vi "ParseServerMessage.vi"(8 "error in (no error)":errorcluster, 10 "msg":string) -> (0 "error out":errorcluster, 2 "ServerFrame":T1)   [LabVIEW 2017, in "LabVIEW STOMP.lvlib" / "STOMP.lvclass"]
uses:
  STOMP.lvclass
  Typedefs/Type_ServerFrame.ctl
  Typedefs/Type_ServerFrameType.ctl
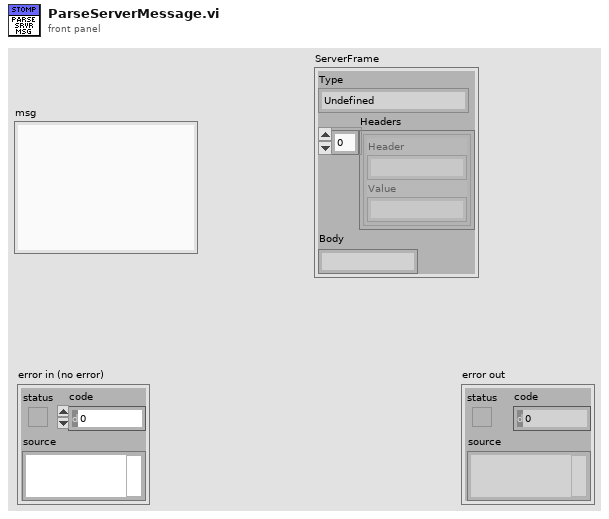
[diagram p1: front panel]
types:
  T1 = typedef "LabVIEW STOMP.lvlib/STOMP.lvclass/Type_ServerFrame.ctl" = cluster{"Type":T2, "Headers":cluster{"Header":string, "Value":string}[], "Body":string}
  T2 = typedef "LabVIEW STOMP.lvlib/STOMP.lvclass/Type_ServerFrameType.ctl" = enum16{"Undefined", "MESSAGE", "CONNECTED", "RECEIPT", "ERROR"}
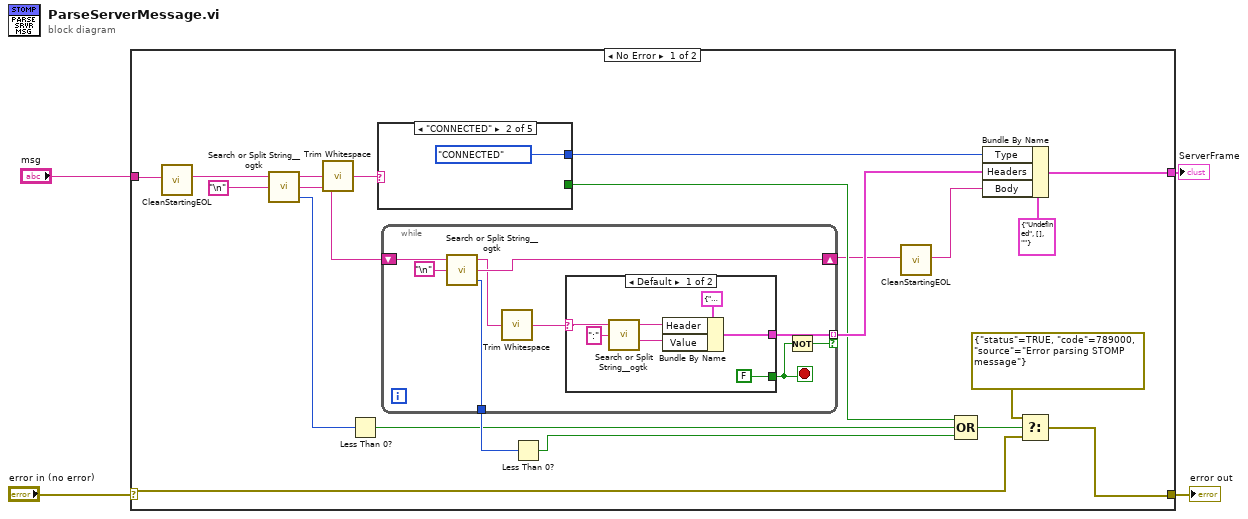
[diagram p0: block diagram]
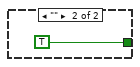
[diagram p2: hidden frame]
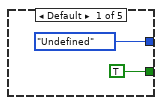
[diagram p3: hidden frame]
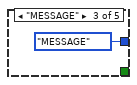
[diagram p4: hidden frame]
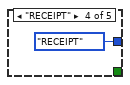
[diagram p5: hidden frame]
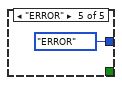
[diagram p6: hidden frame]
diagram:
  n1 = case shown="No Error" "error in (no error)" {
    selector: "error in (no error)" -> [w11 w49]
    tunnel: [w10 w49] -> w3
    tunnel: "msg" -> [w8 _]
    tunnel: [w18 _] -> w1
    frame No Error {
      n2 = call "CleanStartingEOL.vi"("String"=w8) -> ("string"=w7:string)  [unwired: 18 in]
      n3 = call <userlib>:"Search or Split String__ogtk.vi"("search string/char (-)"="\n", "string"=w7) -> ("offset after match"=w17:i32, "substring after match"=w21:string, "substring before match"=w23:string)  [unwired: 1 in]
      n4 = call <vilib>:"Trim Whitespace.vi"("string"=w23) -> ("trimmed string"=w22:string)  [unwired: 1 in]
      n5 = Less Than 0?(x=w17) -> (x < 0?=w15:bool)
      n6 = case shown="\"CONNECTED\"" w22 {
        tunnel: [Type_ServerFrameType."Undefined" ("Type") Type_ServerFrameType."CONNECTED" ("Type") Type_ServerFrameType."MESSAGE" ("Type") Type_ServerFrameType."RECEIPT" ("Type") Type_ServerFrameType."ERROR" ("Type")] -> w19
        tunnel: [TRUE _ _ _ _] -> w13
        frame Default {
        }
        frame "CONNECTED" {
        }
        frame "MESSAGE" {
        }
        frame "RECEIPT" {
        }
        frame "ERROR" {
        }
      }
      n7 = while {
        shift-right: [w32] -> w6
        shift-left: w21 -> [w34]
        tunnel: [w29] -> w20 mode=indexing if=w27
        tunnel: [w26] -> w16
        stop <- w28 stop-if-true
        n8 = call <userlib>:"Search or Split String__ogtk.vi"("search string/char (-)"="\n", "string"=w34) -> ("offset after match"=w26:i32, "substring after match"=w32:string, "substring before match"=w31:string)  [unwired: 1 in]
        n9 = call <vilib>:"Trim Whitespace.vi"("string"=w31) -> ("trimmed string"=w30:string)  [unwired: 1 in]
        n10 = case shown="Default" w30 {
          selector: w30 -> [w40 _]
          tunnel: [FALSE TRUE] -> w28
          tunnel: [w35 _] -> w29
          frame Default {
            n11 = call <userlib>:"Search or Split String__ogtk.vi"("search string/char (-)"=":", "string"=w40) -> ("substring after match"=w36:string, "substring before match"=w37:string)  [unwired: 1 in, 1 out]
            n12 = Bundle By Name(cluster=cluster{"Header":string, "Value":string} {"Header"="", "Value"=""}, "Header"=w37, "Value"=w36) -> (w35:cluster{"Header":string, "Value":string})
          }
          frame "" {
          }
        }
        n13 = Not(x=w28) -> (.not. x?=w27:bool)
      }
      n14 = Less Than 0?(x=w16) -> (x < 0?=w14:bool)
      n15 = call "CleanStartingEOL.vi"("String"=w6) -> ("string"=w5:string)  [unwired: 18 in]
      n16 = Compound Arithmetic op=OR(w13, w15, w14) -> (w12:bool)
      n17 = Bundle By Name(cluster=T1 {"Type"=enum."Undefined", "Headers"=[], "Body"=""}, "Type"=w19, "Headers"=w20, "Body"=w5) -> (w18:T1)
      n18 = Select(t=errorcluster {"status"=TRUE, "code"=789000, "source"="Error parsing STOMP message"} ("error constant"), s=w12, f=w11) -> (s? t:f=w10:errorcluster)
    }
    frame Error {
    }
  }
  "error out" <- w3
  "ServerFrame" <- w1
